vi "AudioStreamer.IsMicDeviceValid.vi"(1 "device":string) -> (0 "result":string)   [LabVIEW 2020]
uses:
  <vilib>/Dataflow_G/G-Audio/G-Audio.lvlib
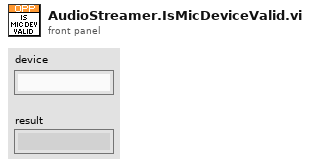
[diagram p1: front panel]
types:
  T1 = typedef "G-Audio.lvlib/Audio Device Info.ctl" = cluster{"Name":string, "ID":u8[], "Device Type":T2, "Default":bool, "Native Data Formats":T3[]}
  T2 = typedef "G-Audio.lvlib/Audio Device Type.ctl" = enum16{"(None)", "Playback", "Capture", "Duplex", "Loopback"}
  T3 = typedef "G-Audio.lvlib/Audio Device Native Data Format.ctl" = cluster{"Format":T4, "Channels":u32, "Sample Rate (Hz)":u32, "Exclusive Mode":bool}
  T4 = typedef "G-Audio.lvlib/Audio Device Format.ctl" = enum16{"Native", "U8", "I16", "I32", "SGL"}
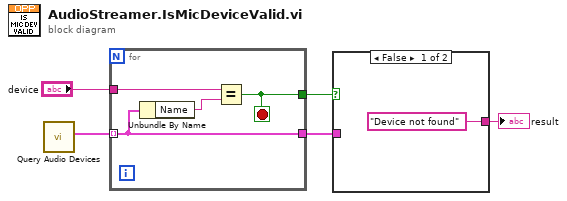
[diagram p0: block diagram]
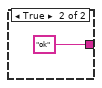
[diagram p2: hidden frame]
diagram:
  n1 = call <vilib>:"Query Audio Devices.vi"() -> ("Capture Devices"=w1:T1[])  [unwired: 7 in, 4 out]
  n2 = for {
    tunnel: w1 -> [w6] mode=indexing
    tunnel: "device" -> [w8]
    tunnel: [w7] -> w3
    tunnel: [w6] -> w4
    stop <- w7 stop-if-true
    n3 = Unbundle By Name(w6) -> ("Name"=w9:string)
    n4 = Equal?(x=w8, y=w9) -> (x = y?=w7:bool)
  }
  n5 = case shown="False" w3 {
    tunnel: w4 -> [_ _]
    tunnel: ["Device not found" "ok"] -> w2
    frame False {
    }
    frame True {
    }
  }
  "result" <- w2
